vi "111_config.vi"() -> ()   [LabVIEW 2020]
uses:
  <vilib>/Utility/config.llb/NI_LVConfig.lvlib
  Global_Variable/Global.vi
  Global_Variable/A131258.vi
panel:
  in  "产品型号":string(combo)
  in  "删除":bool
  in  "确定":bool
  in  "添加":bool
  in  "退出":bool
  in  "更新":bool
  in  "选项卡控件":enum32{"产品参数1", "判定参数", "产品管理"}(tab)
  in  "压销参数":T1
  in  "动力头1参数":T2
  in  "动力头2参数":T2
  in  "移栽轴参数":T3
  in  "系统参数":T4
  in  "力特性参数":T5
  in  "试验项目":cluster{"力特性":bool, "内泄露":bool, "自由间隙":bool}
  in  "定点B(MPa)":dbl
  in  "定点A(MPa)":dbl
  in  "灵敏度":T6
  in  "力特性":T7
  in  "自由间隙(°)":cluster{"下限":dbl, "上限":dbl}
  in  "内泄露(L/Min)":cluster{"下限":dbl, "上限":dbl}
  in  "压力损失(MPa)":cluster{"下限":dbl, "上限":dbl}
  in  "请输入添加的产品名称":string
  in  "请选择要删除的产品":string(combo)
  # "调阀台"
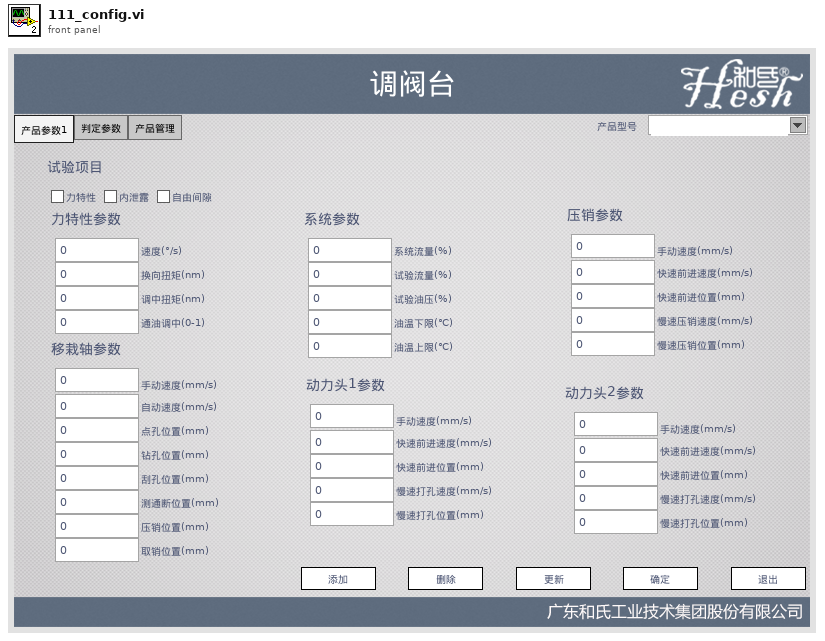
[diagram p1: front panel]
types:
  T1 = cluster{"手动速度(mm/s)":dbl, "快速前进速度(mm/s)":dbl, "快速前进位置(mm)":dbl, "慢速压销速度(mm/s)":dbl, "慢速压销位置(mm)":dbl}
  T2 = cluster{"手动速度(mm/s)":dbl, "快速前进速度(mm/s)":dbl, "快速前进位置(mm)":dbl, "慢速打孔速度(mm/s)":dbl, "慢速打孔位置(mm)":dbl}
  T3 = cluster{"手动速度(mm/s)":dbl, "自动速度(mm/s)":dbl, "点孔位置(mm)":dbl, "钻孔位置(mm)":dbl, "刮孔位置(mm)":dbl, "测通断位置(mm)":dbl, "压销位置(mm)":dbl, "取销位置(mm)":dbl}
  T4 = cluster{"系统流量(%)":dbl, "试验流量(%)":dbl, "试验油压(%)":dbl, "油温下限(℃)":dbl, "油温上限(℃)":dbl}
  T5 = cluster{"速度(°/s)":dbl, "换向扭矩(nm)":dbl, "调中扭矩(nm)":dbl, "通油调中(0-1)":dbl}
  T6 = cluster{"对称性(%)":cluster{"下限":dbl, "上限":dbl}, "正向最大角度(°)":cluster{"下限":dbl, "上限":dbl}, "逆向最大角度(°)":cluster{"下限":dbl, "上限":dbl}}
  T7 = cluster{"对称性(%)":cluster{"下限":dbl, "上限":dbl}, "正向最大油压(MPa)":cluster{"下限":dbl, "上限":dbl}, "逆向最大油压(MPa)":cluster{"下限":dbl, "上限":dbl}, "定点A正向扭矩(Nm)":cluster{"下限":dbl, "上限":dbl}, "定点A逆向扭矩(Nm)":cluster{"上限":dbl, "下限":dbl}, "定点B正向扭矩(Nm)":cluster{"下限":dbl, "上限":dbl}, "定点B逆向扭矩(Nm)":cluster{"下限":dbl, "上限":dbl}}
  T8 = typedef "NI_LVConfig.lvlib/Config Data RefNum.ctl" = refnum<k1>
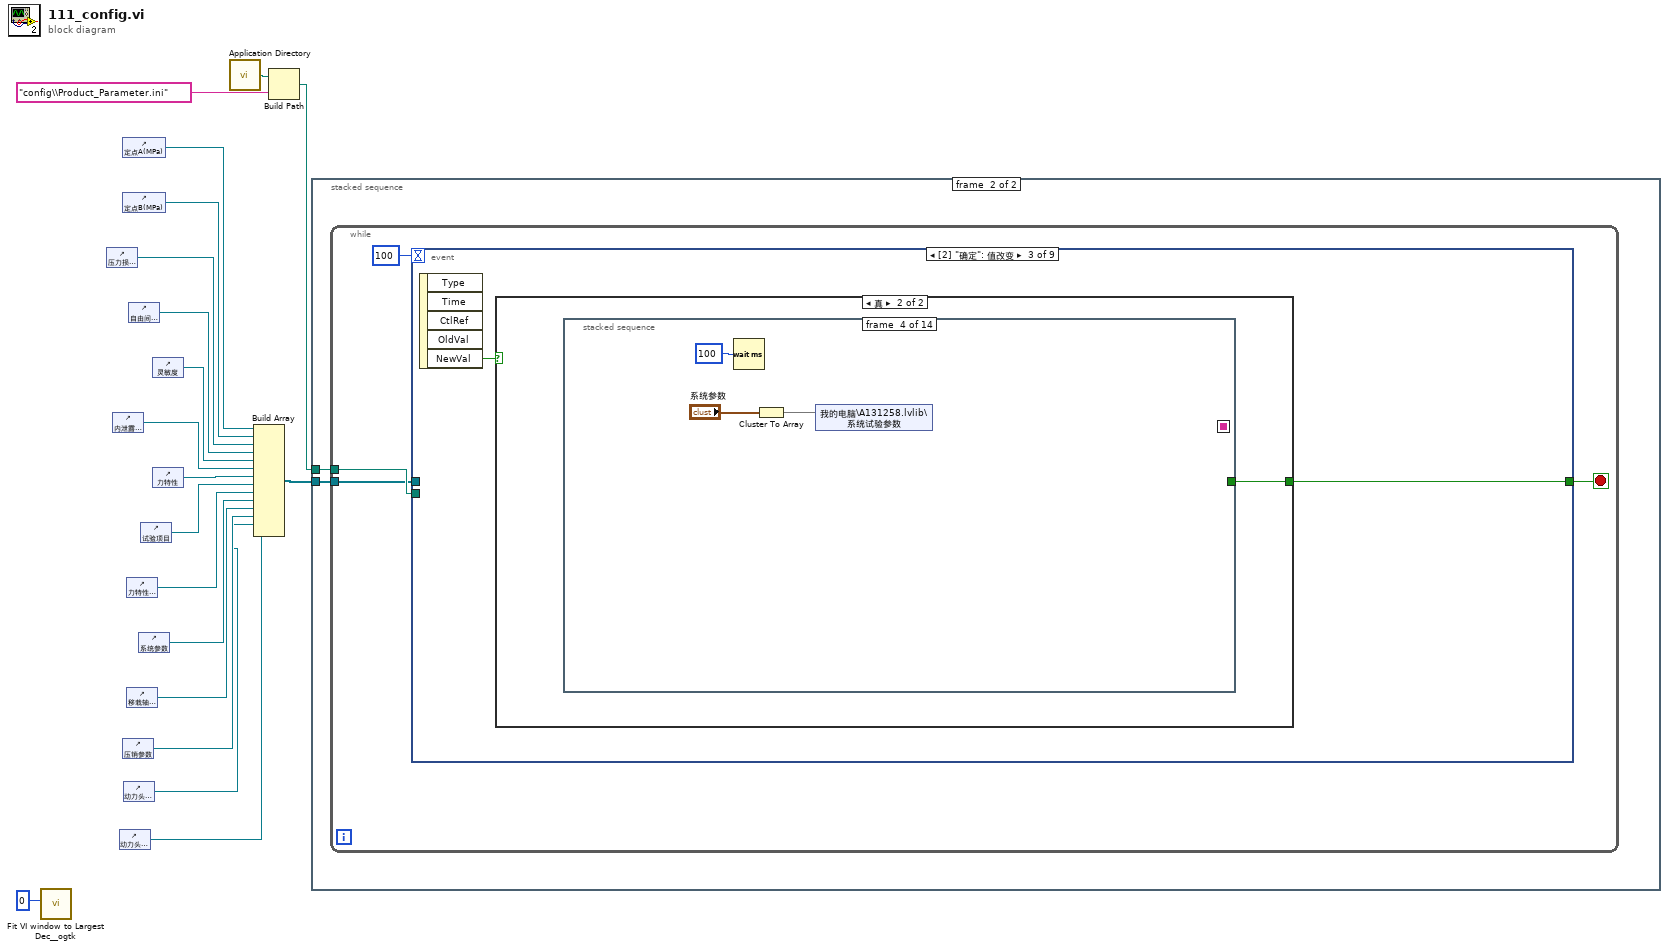
[diagram p0: block diagram]
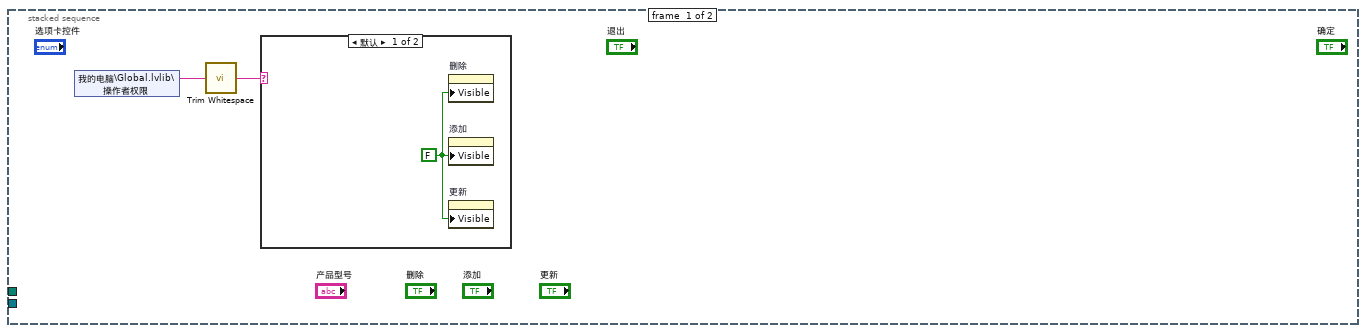
[diagram p2: hidden frame]
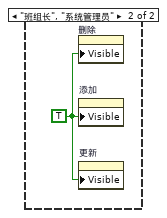
[diagram p3: hidden frame]
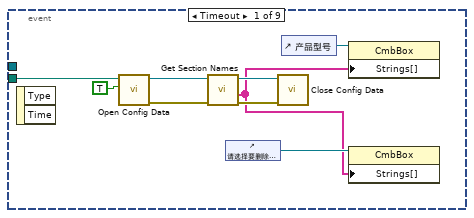
[diagram p4: hidden frame]
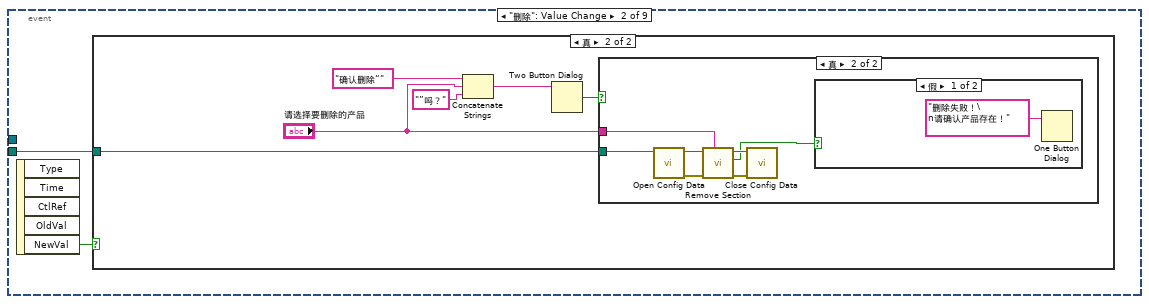
[diagram p5: hidden frame]
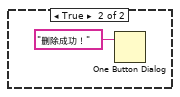
[diagram p8: hidden frame]
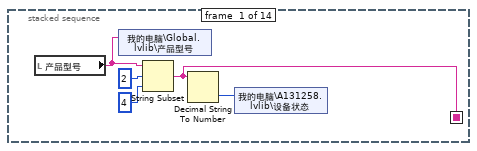
[diagram p10: hidden frame]
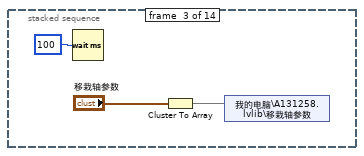
[diagram p12: hidden frame]
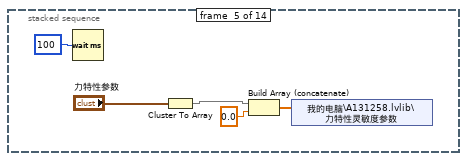
[diagram p13: hidden frame]
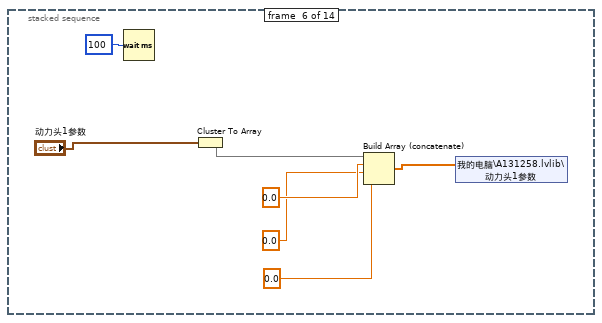
[diagram p14: hidden frame]
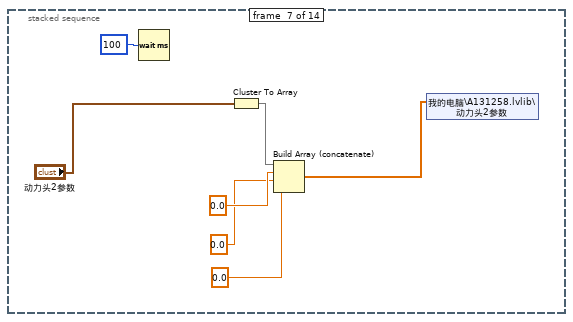
[diagram p15: hidden frame]
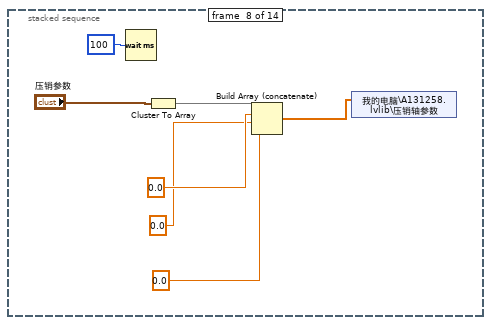
[diagram p16: hidden frame]
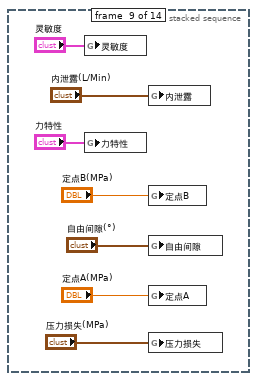
[diagram p17: hidden frame]
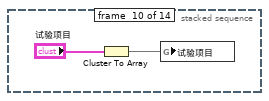
[diagram p18: hidden frame]
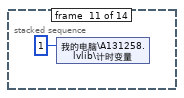
[diagram p19: hidden frame]
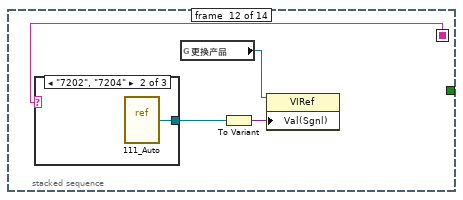
[diagram p20: hidden frame]
diagram:
  n1 = call <userlib>:"Fit VI window to Largest Dec__ogtk.vi"("border spacing (2 px)"=0) -> ()  [unwired: 5 in, 2 out]
  n2 = control-ref of="压力损失(MPa)"() -> (w7:refnum<vi>)
  n3 = control-ref of="内泄露(L/Min)"() -> (w10:refnum<vi>)
  n4 = control-ref of="动力头1参数"() -> (w1:refnum<vi>)
  n5 = control-ref of="定点A(MPa)"() -> (w5:refnum<vi>)
  n6 = control-ref of="定点B(MPa)"() -> (w6:refnum<vi>)
  n7 = control-ref of="压销参数"() -> (w3:refnum<vi>)
  n8 = control-ref of="动力头2参数"() -> (w2:refnum<vi>)
  n9 = control-ref of="力特性参数"() -> (w14:refnum<vi>)
  n10 = control-ref of="移栽轴参数"() -> (w4:refnum<vi>)
  n11 = control-ref of="自由间隙(°)"() -> (w8:refnum<vi>)
  n12 = control-ref of="系统参数"() -> (w13:refnum<vi>)
  n13 = control-ref of="试验项目"() -> (w12:refnum<vi>)
  n14 = control-ref of="灵敏度"() -> (w9:refnum<vi>)
  n15 = control-ref of="力特性"() -> (w11:refnum<vi>)
  n16 = call <vilib>:"Application Directory.vi"() -> ("Application Directory"=w18:path)
  n17 = Build Array(w5, w6, w7, w8, w9, w10, w11, w12, w14, w13, w4, w3, w2, w1) -> (w19:refnum<vi>[])
  n18 = Build Path(base path=w18, name or relative path="config\\Product_Parameter.ini" ("名称或相对路径")) -> (appended path=w16:path)
  n19 = stacked-sequence {
    tunnel: w19 -> [_ w25]
    tunnel: w16 -> [_ w24]
    frame #0 {
      n20 = shared-variable "我的电脑\\Global.lvlib\\操作者权限"() -> (w21:string)  [unwired: 1 in, 1 out]
      n21 = call <vilib>:"Trim Whitespace.vi"("string"=w21) -> ("trimmed string"=w20:string)  [unwired: 1 in]
      n22 = case shown="默认" w20 {
        frame Default {
          w22 = FALSE ("可见")
          n23 = property on="删除" class="Bool (严格)"("Visible"=w22) -> ()  [unwired: 2 in, 2 out]
          n24 = property on="添加" class="Bool (严格)"("Visible"=w22) -> ()  [unwired: 2 in, 2 out]
          n25 = property on="更新" class="Bool (严格)"("Visible"=w22) -> ()  [unwired: 2 in, 2 out]
        }
        frame "班组长", "系统管理员" {
          w23 = TRUE ("可见")
          n26 = property on="删除" class="Bool (严格)"("Visible"=w23) -> ()  [unwired: 2 in, 2 out]
          n27 = property on="添加" class="Bool (严格)"("Visible"=w23) -> ()  [unwired: 2 in, 2 out]
          n28 = property on="更新" class="Bool (严格)"("Visible"=w23) -> ()  [unwired: 2 in, 2 out]
        }
      }
    }
    frame #1 {
      n29 = while {
        tunnel: w24 -> [w29]
        tunnel: w25 -> [w27]
        stop <- w28 stop-if-true
        n30 = event shown="[2] \"确定\": 值改变" {
          selector: _ -> [_ _ _ _ _ _ _ _ _]
          dyn-events: _ -> [_ _ _ _ _ _ _ _ _]
          timeout: 100 -> [_ _ _ _ _ _ _ _ _]
          tunnel: w29 -> [w33 w40 _ w120 w135 _ w149 _ _]
          tunnel: [_ _ w56 _ _ TRUE _ _ TRUE] -> w28
          tunnel: w27 -> [_ _ _ w121 w136 _ w148 _ _]
          event Timeout {
            n31 = event-data() -> ()  [unwired: 1 in, 2 out]
            n32 = call <vilib>:"Open Config Data.vi"("create file if necessary (T)"=TRUE, "configuration file path"=w33) -> ("error out"=w35:errorcluster, "refnum"=w34:T8)  [unwired: 7 in, 1 out]
            n33 = call <vilib>:"Get Section Names.vi"("error in (no error)"=w35, "refnum"=w34) -> ("error out"=w37:errorcluster, "section names"=w30:string[], "refnum out"=w36:T8)  [unwired: 7 in]
            n34 = control-ref of="请选择要删除的产品"() -> (w31:refnum<vi>)
            n35 = call <vilib>:"Close Config Data.vi"("error in (no error)"=w37, "refnum"=w36) -> ()  [unwired: 8 in, 2 out]
            n36 = control-ref of="产品型号"() -> (w32:refnum<vi>)
            n37 = property on="属性节点" class="CmbBox"(reference=w32, "Strings[]"=w30) -> ()  [unwired: 1 in, 2 out]
            n38 = property on="属性节点" class="CmbBox"(reference=w31, "Strings[]"=w30) -> ()  [unwired: 1 in, 2 out]
          }
          event "删除": Value Change {
            n39 = event-data() -> ("NewVal"=w39:bool)  [unwired: 1 in, 4 out]
            n40 = case shown="真" w39 {
              tunnel: w40 -> [_ w42]
              frame False {
              }
              frame True {
                n41 = Concatenate Strings("确认删除“", "请选择要删除的产品", "”吗？") -> (w44:string)
                n42 = Two Button Dialog(message=w44) -> (T button?=w43:bool)  [unwired: 2 in]
                n43 = case shown="真" w43 {
                  tunnel: w42 -> [_ w48]
                  tunnel: "请选择要删除的产品" -> [_ w47]
                  frame False {
                  }
                  frame True {
                    n44 = call <vilib>:"Open Config Data.vi"("configuration file path"=w48) -> ("error out"=w50:errorcluster, "refnum"=w53:T8)  [unwired: 8 in, 1 out]
                    n45 = call <vilib>:"Remove Section.vi"("section"=w47, "error in (no error)"=w50, "refnum"=w53) -> ("error out"=w52:errorcluster, "section exists?"=w49:bool, "refnum out"=w51:T8)  [unwired: 6 in]
                    n46 = call <vilib>:"Close Config Data.vi"("error in (no error)"=w52, "refnum"=w51) -> ()  [unwired: 8 in, 2 out]
                    n47 = case shown="假" w49 {
                      frame False {
                        n48 = One Button Dialog(message="删除失败！\n请确认产品存在！" ("消息")) -> ()  [unwired: 1 in, 1 out]
                      }
                      frame True {
                        n49 = One Button Dialog(message="删除成功！" ("消息")) -> ()  [unwired: 1 in, 1 out]
                      }
                    }
                  }
                }
              }
            }
          }
          event "确定": Value Change {
            n50 = event-data() -> ("NewVal"=w57:bool)  [unwired: 1 in, 4 out]
            n51 = case shown="真" w57 {
              tunnel: [_ w58] -> w56
              frame False {
              }
              frame True {
                n52 = stacked-sequence {
                  seq-local: [w63 _ _ _ _ _ _ _ _ _ _ _ _ _] -> [_ _ _ _ _ _ _ _ _ _ _ w109 _ _]
                  tunnel: [_ _ _ _ _ _ _ _ _ _ _ _ _ TRUE] -> w58
                  frame #0 {
                    n53 = local read "产品型号"() -> (w62:string)
                    n54 = shared-variable "我的电脑\\Global.lvlib\\产品型号"(w62) -> ()  [unwired: 1 in, 1 out]
                    n55 = String Subset(string=w62, offset (0)=u16 2 ("偏移量(0)"), length (rest)=u16 4 ("长度（剩余）")) -> (substring=w63:string)
                    n56 = Decimal String To Number(string=w63) -> (number=w59:i32)  [unwired: 2 in, 1 out]
                    n57 = shared-variable "我的电脑\\A131258.lvlib\\设备状态"(w59) -> ()  [unwired: 1 in, 1 out]
                  }
                  frame #1 {
                  }
                  frame #2 {
                    n58 = Wait (ms)(milliseconds to wait=u32 100 ("等待时间（毫秒）")) -> ()  [unwired: 1 out]
                    n59 = Cluster To Array(cluster="移栽轴参数") -> (array=w65:dbl[])
                    n60 = shared-variable "我的电脑\\A131258.lvlib\\移栽轴参数"(w65) -> ()  [unwired: 1 in, 1 out]
                  }
                  frame #3 {
                    n61 = Wait (ms)(milliseconds to wait=u32 100 ("等待时间（毫秒）")) -> ()  [unwired: 1 out]
                    n62 = Cluster To Array(cluster="系统参数") -> (array=w68:dbl[])
                    n63 = shared-variable "我的电脑\\A131258.lvlib\\系统试验参数"(w68) -> ()  [unwired: 1 in, 1 out]
                  }
                  frame #4 {
                    n64 = Wait (ms)(milliseconds to wait=u32 100 ("等待时间（毫秒）")) -> ()  [unwired: 1 out]
                    n65 = Cluster To Array(cluster="力特性参数") -> (array=w73:dbl[])
                    n66 = Build Array (concatenate)(w73, sgl 0.0) -> (w72:dbl[])
                    n67 = shared-variable "我的电脑\\A131258.lvlib\\力特性灵敏度参数"(w72) -> ()  [unwired: 1 in, 1 out]
                  }
                  frame #5 {
                    n68 = Wait (ms)(milliseconds to wait=u32 100 ("等待时间（毫秒）")) -> ()  [unwired: 1 out]
                    n69 = Cluster To Array(cluster="动力头1参数") -> (array=w79:dbl[])
                    n70 = Build Array (concatenate)(w79, sgl 0.0, sgl 0.0, sgl 0.0) -> (w75:dbl[])
                    n71 = shared-variable "我的电脑\\A131258.lvlib\\动力头1参数"(w75) -> ()  [unwired: 1 in, 1 out]
                  }
                  frame #6 {
                    n72 = Wait (ms)(milliseconds to wait=u32 100 ("等待时间（毫秒）")) -> ()  [unwired: 1 out]
                    n73 = Cluster To Array(cluster="动力头2参数") -> (array=w86:dbl[])
                    n74 = Build Array (concatenate)(w86, sgl 0.0, sgl 0.0, sgl 0.0) -> (w85:dbl[])
                    n75 = shared-variable "我的电脑\\A131258.lvlib\\动力头2参数"(w85) -> ()  [unwired: 1 in, 1 out]
                  }
                  frame #7 {
                    n76 = Wait (ms)(milliseconds to wait=u32 100 ("等待时间（毫秒）")) -> ()  [unwired: 1 out]
                    n77 = Cluster To Array(cluster="压销参数") -> (array=w90:dbl[])
                    n78 = Build Array (concatenate)(w90, sgl 0.0, sgl 0.0, sgl 0.0) -> (w89:dbl[])
                    n79 = shared-variable "我的电脑\\A131258.lvlib\\压销轴参数"(w89) -> ()  [unwired: 1 in, 1 out]
                  }
                  frame #8 {
                    n80 = global write "A131258.vi" "灵敏度"("灵敏度") -> ()
                    n81 = global write "A131258.vi" "力特性"("力特性") -> ()
                    n82 = global write "A131258.vi" "内泄露"("内泄露(L/Min)") -> ()
                    n83 = global write "A131258.vi" "定点B"("定点B(MPa)") -> ()
                    n84 = global write "A131258.vi" "自由间隙"("自由间隙(°)") -> ()
                    n85 = global write "A131258.vi" "定点A"("定点A(MPa)") -> ()
                    n86 = global write "A131258.vi" "压力损失"("压力损失(MPa)") -> ()
                  }
                  frame #9 {
                    n87 = Cluster To Array(cluster="试验项目") -> (array=w103:bool[])
                    n88 = global write "Global.vi" "试验项目"(w103) -> ()
                  }
                  frame #10 {
                    n89 = shared-variable "我的电脑\\A131258.lvlib\\计时变量"(u16 1 ("计时变量")) -> ()  [unwired: 1 in, 1 out]
                  }
                  frame #11 {
                    n90 = case shown="\"7202\", \"7204\"" w109 {
                      tunnel: [w110 w111 w112] -> w106
                      frame Default {
                        n91 = vi-ref "111_Auto.vi"() -> (w110:refnum<vi>)
                      }
                      frame "7202", "7204" {
                        n92 = vi-ref "111_Auto.vi"() -> (w111:refnum<vi>)
                      }
                      frame "7205" {
                        n93 = vi-ref "111_Auto.vi"() -> (w112:refnum<vi>)
                      }
                    }
                    n94 = global read "Global.vi" "更换产品"() -> (w108:refnum<vi>)
                    n95 = To Variant(anything=w106) -> (Variant=w107:variant)
                    n96 = property class="VIRef"(reference=w108, "Val(Sgnl)"=w107) -> ()  [unwired: 1 in, 2 out]
                  }
                  frame #12 {
                    w113 = "参数装载成功！" ("消息")
                    n97 = call "浮动通知.vi"("通知内容"=w113) -> ()  [unwired: 11 in]
                    n98 = One Button Dialog(message=w113) -> ()  [unwired: 1 in, 1 out]
                  }
                  frame #13 {
                    n99 = control-ref of="本VI"() -> (w115:refnum<vi>)
                    n100 = invoke class="VI" method="FP.Close"(reference=w115) -> ()  [unwired: 2 in, 3 out]
                  }
                }
              }
            }
          }
          event "添加": Value Change {
            n101 = event-data() -> ("NewVal"=w119:bool)  [unwired: 1 in, 4 out]
            n102 = local read "请输入添加的产品名称"() -> (w118:string)
            n103 = call <vilib>:"Trim Whitespace.vi"("string"=w118) -> ("trimmed string"=w116:string)  [unwired: 1 in]
            n104 = White Space?(1:w116) -> (0:w117:bool)
            n105 = case shown="假" w117 {
              tunnel: w121 -> [w124 _]
              tunnel: w120 -> [w123 _]
              tunnel: w119 -> [w122 _]
              frame False {
                n106 = case shown="真" w122 {
                  tunnel: w124 -> [_ w126]
                  tunnel: w123 -> [_ w125]
                  frame False {
                  }
                  frame True {
                    n107 = for {
                      tunnel: w126 -> [w128] mode=indexing
                      tunnel: w125 -> [w127]
                      n108 = call "Read_Write ParaINI File.vi"("Mode"=enum16{"Read", "Write"}."Write", "Section"="请输入添加的产品名称", "Filepath"=w127, "Ctl Refnum"=w128) -> ()  [unwired: 7 in, 1 out]
                    }
                  }
                }
              }
              frame True {
                w131 = 64 items=["None"=0, "Hand, Error, Stop"=16, "Question"=32, "Exclamation, Warning"=48, "Asterisk, Information"=64] ("icon")
                w132 = 0 items=["OK", "OKCancel", "AbortRetryIgnore", "YesNoCancel", "YesNo", "RetryCancel"] ("buttons")
                n109 = call "信息框（标题、文本、图标）.vi"("icon"=w131, "buttons"=w132, "caption"="添加失败", "text"="请输入产品名称!") -> ()  [unwired: 6 in, 2 out]
              }
            }
          }
          event "产品型号": Value Change {
            n110 = event-data() -> ()  [unwired: 1 in, 5 out]
            n111 = stacked-sequence {
              tunnel: w136 -> [_ w138]
              tunnel: w135 -> [_ w137]
              frame #0 {
              }
              frame #1 {
                n112 = for {
                  tunnel: w138 -> [w141] mode=indexing
                  tunnel: w137 -> [w140]
                  n113 = local read "产品型号"() -> (w139:string)
                  n114 = call "Read_Write ParaINI File.vi"("Mode"=enum16{"Read", "Write"}."Read", "Section"=w139, "Filepath"=w140, "Ctl Refnum"=w141) -> ()  [unwired: 7 in, 1 out]
                }
              }
            }
          }
          event "退出": Value Change {
            n115 = event-data() -> ()  [unwired: 1 in, 5 out]
            n116 = control-ref of="本VI"() -> (w145:refnum<vi>)
            n117 = invoke class="VI" method="FP.Close"(reference=w145) -> (reference out=w143:refnum<vi>, error out=w144:errorcluster)  [unwired: 2 in, 1 out]
            n118 = Close Reference(reference=w143, error in (no error)=w144) -> ()  [unwired: 1 out]
          }
          event "更新": Value Change {
            n119 = event-data() -> ("NewVal"=w147:bool)  [unwired: 1 in, 4 out]
            n120 = case shown="真" w147 {
              tunnel: w149 -> [_ w152]
              tunnel: w148 -> [_ w151]
              frame False {
              }
              frame True {
                n121 = for {
                  tunnel: w152 -> [w157]
                  tunnel: w151 -> [w156] mode=indexing
                  tunnel: [w155] -> w150
                  n122 = local read "产品型号"() -> (w159:string)
                  n123 = call "Read_Write ParaINI File.vi"("Mode"=enum16{"Read", "Write"}."Write", "Section"=w159, "Filepath"=w157, "Ctl Refnum"=w156) -> ("error out"=w155:errorcluster)  [unwired: 7 in]
                }
                n124 = case shown="错误" w150 {
                  frame No Error {
                    n125 = call "浮动通知.vi"("通知内容"="更新成功！") -> ()  [unwired: 11 in]
                  }
                  frame Error {
                    n126 = call "浮动通知.vi"("通知内容"="更新失败！") -> ()  [unwired: 11 in]
                  }
                }
              }
            }
          }
          event "请输入添加的产品名称": Value Change {
            n127 = event-data() -> ("NewVal"=w162:string)  [unwired: 1 in, 4 out]
            n128 = control-ref of="产品型号"() -> (w160:refnum<vi>)
            n129 = property on="属性节点" class="CmbBox"(reference=w160) -> ("Strings[]"=w161:string[])  [unwired: 1 in, 2 out]
            n130 = for {
              tunnel: w162 -> [w163]
              tunnel: w161 -> [w164] mode=indexing
              n131 = Equal?(x=w163, y=w164) -> (x = y?=w165:bool)
              n132 = case shown="真" w165 {
                tunnel: w163 -> [_ w166]
                frame False {
                }
                frame True {
                  n133 = stacked-sequence {
                    tunnel: w166 -> [w172 _]
                    frame #0 {
                      w167 = 64 items=["None"=0, "Hand, Error, Stop"=16, "Question"=32, "Exclamation, Warning"=48, "Asterisk, Information"=64] ("icon")
                      w168 = 0 items=["OK", "OKCancel", "AbortRetryIgnore", "YesNoCancel", "YesNo", "RetryCancel"] ("buttons")
                      n134 = Concatenate Strings("已经存在产品”" ("text"), w172, "“\n请勿重复添加！" ("字符串")) -> (w170:string)
                      n135 = call "信息框（标题、文本、图标）.vi"("icon"=w167, "buttons"=w168, "caption"="产品重复", "text"=w170) -> ()  [unwired: 6 in, 2 out]
                    }
                    frame #1 {
                      n136 = local write "请输入添加的产品名称"("" ("请输入添加的产品名称")) -> ()
                    }
                  }
                }
              }
            }
          }
          event Panel Close {
            n137 = event-data() -> ()  [unwired: 1 in, 3 out]
          }
        }
      }
    }
  }
